vi "Configure Generator ARB File.vi"(8 "error in (no error)":errorcluster, 9 "File Name (\"\")":string, 10 "Instance (1)":i32=1 format="%.0g", 11 "VISA resource name":refnum<visa-resource-name>) -> (0 "error out":errorcluster, 3 "VISA resource name out":refnum<visa-resource-name>)   [LabVIEW 2015, in "Rohde&Schwarz CMXP GPRF.lvlib"]
doc: "Selects a waveform file, to be used for the arbitrary waveform generator.\n\nAttribute:\nRSCMXPGPRF_ATTR_ARB_FILE\n\nRemote-control command:\nSOURce:GPRF:GEN<i>:ARB:FILE"
uses:
  <instrlib>/Rohde&Schwarz CMXP GPRF/Rohde&Schwarz CMXP GPRF.lvlib
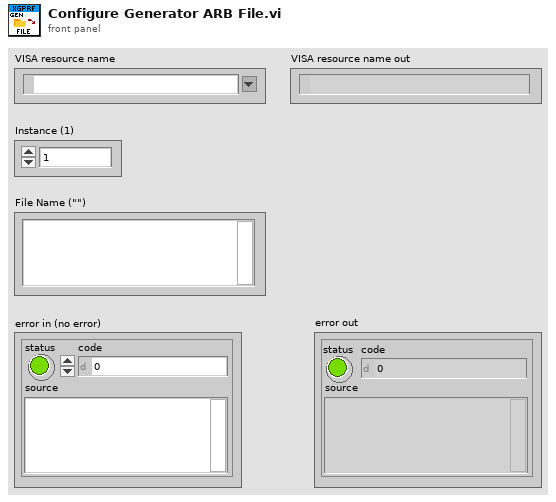
[diagram p1: front panel]
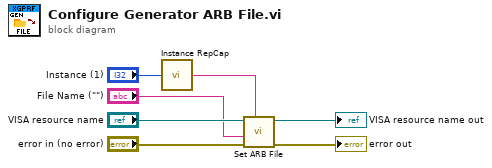
[diagram p0: block diagram]
diagram:
  n1 = call <instrlib>:"Instance RepCap.vi"("instance  in"="Instance (1)") -> ("instance out"=w2:string)
  n2 = call "Set ARB File"("Repeated Capabilities"=w2, "error in (no error)"="error in (no error)", "ARB File ()"="File Name (\"\")", "instrument handle"="VISA resource name") -> ("error out"=→"error out":errorcluster, "instrument handle out"=→"VISA resource name out":refnum<visa-resource-name>)  [unwired: 6 in]
